vi "Remove.vi"(8 "error in (no error)":errorcluster, 9 "ms Timeout (500)":u32=500, 10 "Timer Message":string, 11 "Queue in":refnum<queue>) -> (0 "error out":errorcluster, 2 "Found?":bool, 3 "Queue out":refnum<queue>)   [LabVIEW 2018, in "QueueTimer.lvlib"]
doc: "Remove a queue timer. This stops the timer and waits for the daemon to close.\n\nNote: The Wait on Async timeout is hardcoded that supports to following timout values: 0ms (No wait), 500ms, 2000ms and 5000ms."
uses:
  QueueTimer.lvlib
  <vilib>/ErrorRing/Error Ring.xnode
  <vilib>/Utility/error.llb/Error Cluster From Error Code.vi
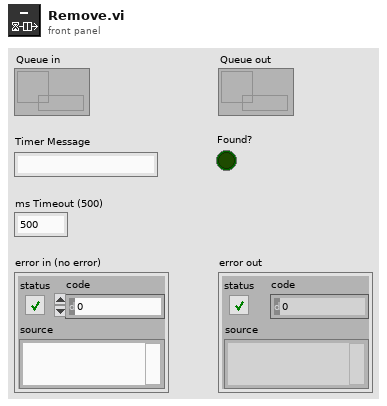
[diagram p1: front panel]
types:
  T1 = cluster{"Emit":refnum<queue>, "Time":refnum<data-value>, "Daemon":refnum<vi>}
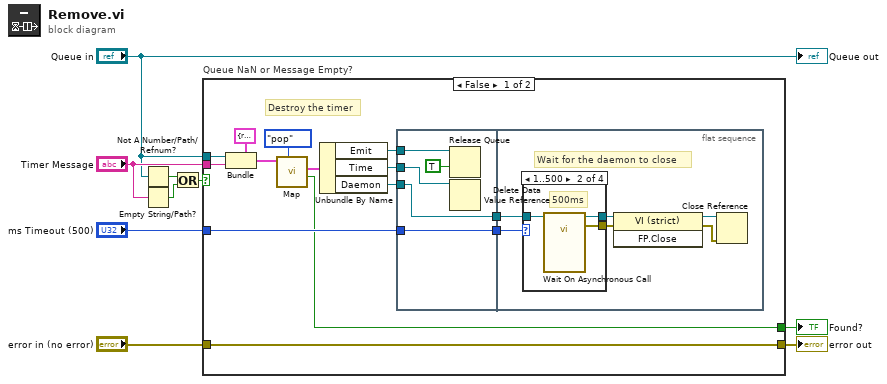
[diagram p0: block diagram]
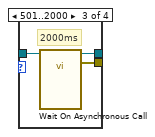
[diagram p3: hidden frame]
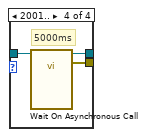
[diagram p4: hidden frame]
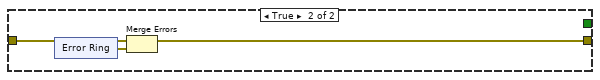
[diagram p5: hidden frame]
diagram:
  n1 = Not A Number/Path/Refnum?(number/path/refnum="Queue in") -> (NaN/Path/Refnum?=w8:bool)
  n2 = Empty String/Path?(string/path="Timer Message") -> (empty?=w9:bool)
  n3 = Or(x=w8, y=w9) -> (x .or. y?=w5:bool)
  n4 = case "Queue NaN or Message Empty?" shown="False" w5 {
    tunnel: "Queue in" -> [w16 _]
    tunnel: "Timer Message" -> [w15 _]
    tunnel: "error in (no error)" -> [w18 w47]
    tunnel: [w18 w46] -> w6
    tunnel: "ms Timeout (500)" -> [w11 _]
    tunnel: [w10 _] -> w1
    frame False {
      # "Destroy the timer"
      n5 = Bundle(cluster=cluster{"Queue":refnum<queue>, "Message":string} {"Queue"=refnum, "Message"=""} ("Timer Id"), "Queue"=w16, "Message"=w15) -> (w17:cluster{"Queue":refnum<queue>, "Message":string})
      n6 = call "Map.vi"("Action"=enum8{"noop", "get", "set", "pop"}."pop", "Timer Id"=w17) -> ("Found?"=w10:bool, "Timer out"=w22:T1)  [unwired: 8 in]
      n7 = Unbundle By Name(w22) -> ("Emit"=w20:refnum<queue>, "Time"=w19:refnum<data-value>, "Daemon"=w14:refnum<vi>)
      n8 = flat-sequence {
        tunnel: w20 -> [w28]
        tunnel: w19 -> [w26]
        tunnel: w14 -> [w25]
        tunnel: [w25] -> w13
        tunnel: [w24] -> w12
        tunnel: w11 -> [w24]
        tunnel: w13 -> [w34]
        tunnel: w12 -> [w29]
        frame #0 {
          n9 = Release Queue(queue=w28, force destroy? (F)=TRUE) -> ()  [unwired: 1 in, 3 out]
          n10 = Delete Data Value Reference(data value reference=w26) -> ()  [unwired: 1 in, 2 out]
        }
        frame #1 {
          # "Wait for the daemon to close"
          n11 = case shown="1..500" w29 {
            tunnel: w34 -> [w35 w38 w41 w44]
            tunnel: [w35 w37 w40 w43] -> w33
            tunnel: [_ w36 w39 w42] -> w32
            frame 0 {
            }
            frame 1..500 {
              # "500ms"
              n12 = call-by-ref "Wait On Asynchronous Call"(reference=w38) -> (reference out=w37:refnum<vi>, error out=w36:errorcluster)  [unwired: 13 in]
            }
            frame 501..2000 {
              # "2000ms"
              n13 = call-by-ref "Wait On Asynchronous Call"(reference=w41) -> (reference out=w40:refnum<vi>, error out=w39:errorcluster)  [unwired: 13 in]
            }
            frame 2001.. {
              # "5000ms"
              n14 = call-by-ref "Wait On Asynchronous Call"(reference=w44) -> (reference out=w43:refnum<vi>, error out=w42:errorcluster)  [unwired: 13 in]
            }
          }
          n15 = invoke class="VI (strict)" method="FP.Close"(reference=w33, error in=w32) -> (reference out=w31:refnum<vi>, error out=w30:errorcluster)  [unwired: 1 in, 1 out]
          n16 = Close Reference(reference=w31, error in (no error)=w30) -> ()  [unwired: 1 out]
        }
      }
    }
    frame True {
      n17 = xnode "Error Ring"() -> ("error out"=w45:errorcluster)
      n18 = Merge Errors(w47, w45) -> (w46:errorcluster)
    }
  }
  "error out" <- w6
  "Found?" <- w1
  "Queue out" <- "Queue in"
